vi "Create Action Point.vi"(8 "error in":errorcluster, 10 "Action Point Identifier":string) -> (0 "error out":errorcluster, 2 "IAction Point out":refnum<class "Action Point.lvclass">)   [LabVIEW 2024, in "Instrument Manager.lvclass"]
uses:
  Instrument Manager.lvclass
  Config from JSON/Config from JSON.lvclass
  Instrument Manager.lvclass/Instrument Manager.ctl
  Action Point/Action Point.lvclass
  Interfaces/IVirtual Instrument/IVirtual Instrument.lvclass
  D:/git/HAL/Source/Config from JSON/Config from JSON.lvclass
  D:/git/HAL/Source/Interfaces/IConfiguration/IConfiguration.lvclass
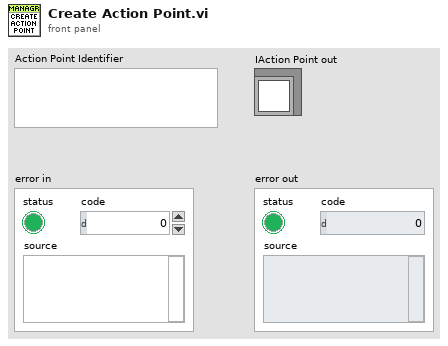
[diagram p1: front panel]
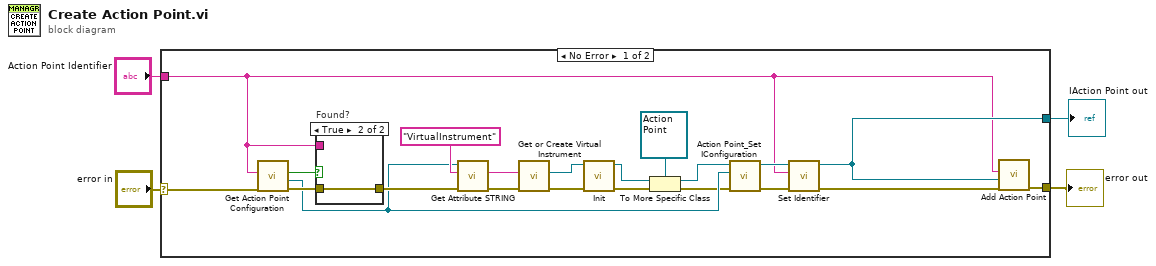
[diagram p0: block diagram]
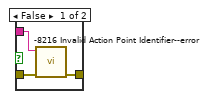
[diagram p2: hidden frame]
diagram:
  n1 = case shown="No Error" "error in" {
    selector: "error in" -> [w15 w28]
    tunnel: [w22 w28] -> w3
    tunnel: "Action Point Identifier" -> [w8 _]
    tunnel: [w9 _] -> w1
    frame No Error {
      n2 = call "Get Action Point Configuration.vi"("Error In"=w15, "Action Point Configuration"=w8) -> ("Error Out"=w20:errorcluster, "Config from JSON"=w13:refnum<class "Config from JSON.lvclass">, "Found"=w21:bool)  [unwired: 7 in]
      n3 = case "Found?" shown="True" w21 {
        tunnel: w20 -> [w26 w27]
        tunnel: [w25 w27] -> w19
        tunnel: w8 -> [w24 _]
        frame False {
          n4 = call "-8216 Invalid Action Point Identifier--error.vi"("error in"=w26, "Source"=w24) -> ("error out"=w25:errorcluster)  [unwired: 9 in]
        }
        frame True {
        }
      }
      n5 = call-dynamic "Get Attribute STRING.vi"("error in"=w19, "Attribute"="VirtualInstrument", "ConfigFromJSON in"=w13) -> ("error out"=w16:errorcluster, "Value"=w11:string)  [unwired: 6 in, 1 out]
      n6 = call "Get or Create Virtual Instrument.vi"("Error In"=w16, "Virtual Instrument Identifier"=w11) -> ("Error Out"=w12:errorcluster, "IVritual Instrument"=w6:refnum<class "IVirtual Instrument.lvclass">)  [unwired: 8 in]
      n7 = call-dynamic "Init.vi"("error in"=w12, "IInitialize in"=w6) -> ("error out"=w7:errorcluster, "IInitialize out"=w5:refnum<class "IVirtual Instrument.lvclass">)  [unwired: 8 in]
      n8 = To More Specific Class(target class=refnum<class "Action Point.lvclass"> refnum ("Action Point.lvclass"), reference=w5, error in=w7) -> (specific class reference=w18:refnum<class "Action Point.lvclass">, error out=w10:errorcluster)
      n9 = call "Action Point_Set IConfiguration.vi"("IConfiguration"=w13, "Action Point in"=w18) -> ("Action Point out"=w14:refnum<class "Action Point.lvclass">)  [unwired: 9 in]
      n10 = call "Set Identifier.vi"("Identifier"=w8, "Action Point in"=w14) -> ("Action Point out"=w9:refnum<class "Action Point.lvclass">)  [unwired: 9 in]
      n11 = call "Add Action Point.vi"("Error In"=w10, "Action Point"=w9, "Action Point Identifier"=w8) -> ("Error Out"=w22:errorcluster)  [unwired: 8 in]
    }
    frame Error {
    }
  }
  "error out" <- w3
  "IAction Point out" <- w1
